vi "search instance list for class.vi"(10 "UID":string, 11 "instance data":T1[](array[typedef])) -> (3 "index":i32)   [LabVIEW 2013, in "NISE_CEF_TreeSerializer.lvlib"]
doc: "Searches a flattened instance set for a given class and returns the index of the first match."
uses:
  NISE_CEF_TreeSerializer.lvlib
  instance data.ctl
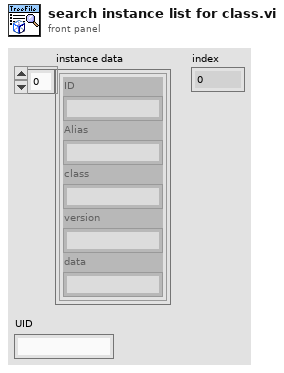
[diagram p1: front panel]
types:
  T1 = typedef "NISE_CEF_TreeSerializer.lvlib/instance data.ctl" = cluster{"ID":string, "Alias":string, "class":string, "version":string, "data":string}
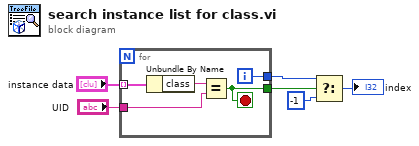
[diagram p0: block diagram]
diagram:
  n1 = for {
    tunnel: "instance data" -> [w8] mode=indexing
    tunnel: "UID" -> [w11]
    tunnel: [w10] -> w5
    tunnel: [w9] -> w6
    i -> [w10]
    stop <- w9 stop-if-true
    n2 = Unbundle By Name(w8) -> ("class"=w7:string)
    n3 = Equal?(x=w7, y=w11) -> (x = y?=w9:bool)
  }
  n4 = Select(t=w5, s=w6, f=-1) -> (s? t:f=→"index":i32)
